vi "Improved find target.vi"(9 "robot location":dbl[](array[numeric]), 10 "Dispaly map":u16[][](array[ring])) -> (2 "target location":dbl[](array[numeric]))   [LabVIEW 2015]
panel:
  out "points":dbl
  out "Highest priority locations":i32[][](array[numeric])
  out "distances":dbl[](array[numeric])
  out "Priority map":dbl[][](array[numeric])
  out "x":dbl
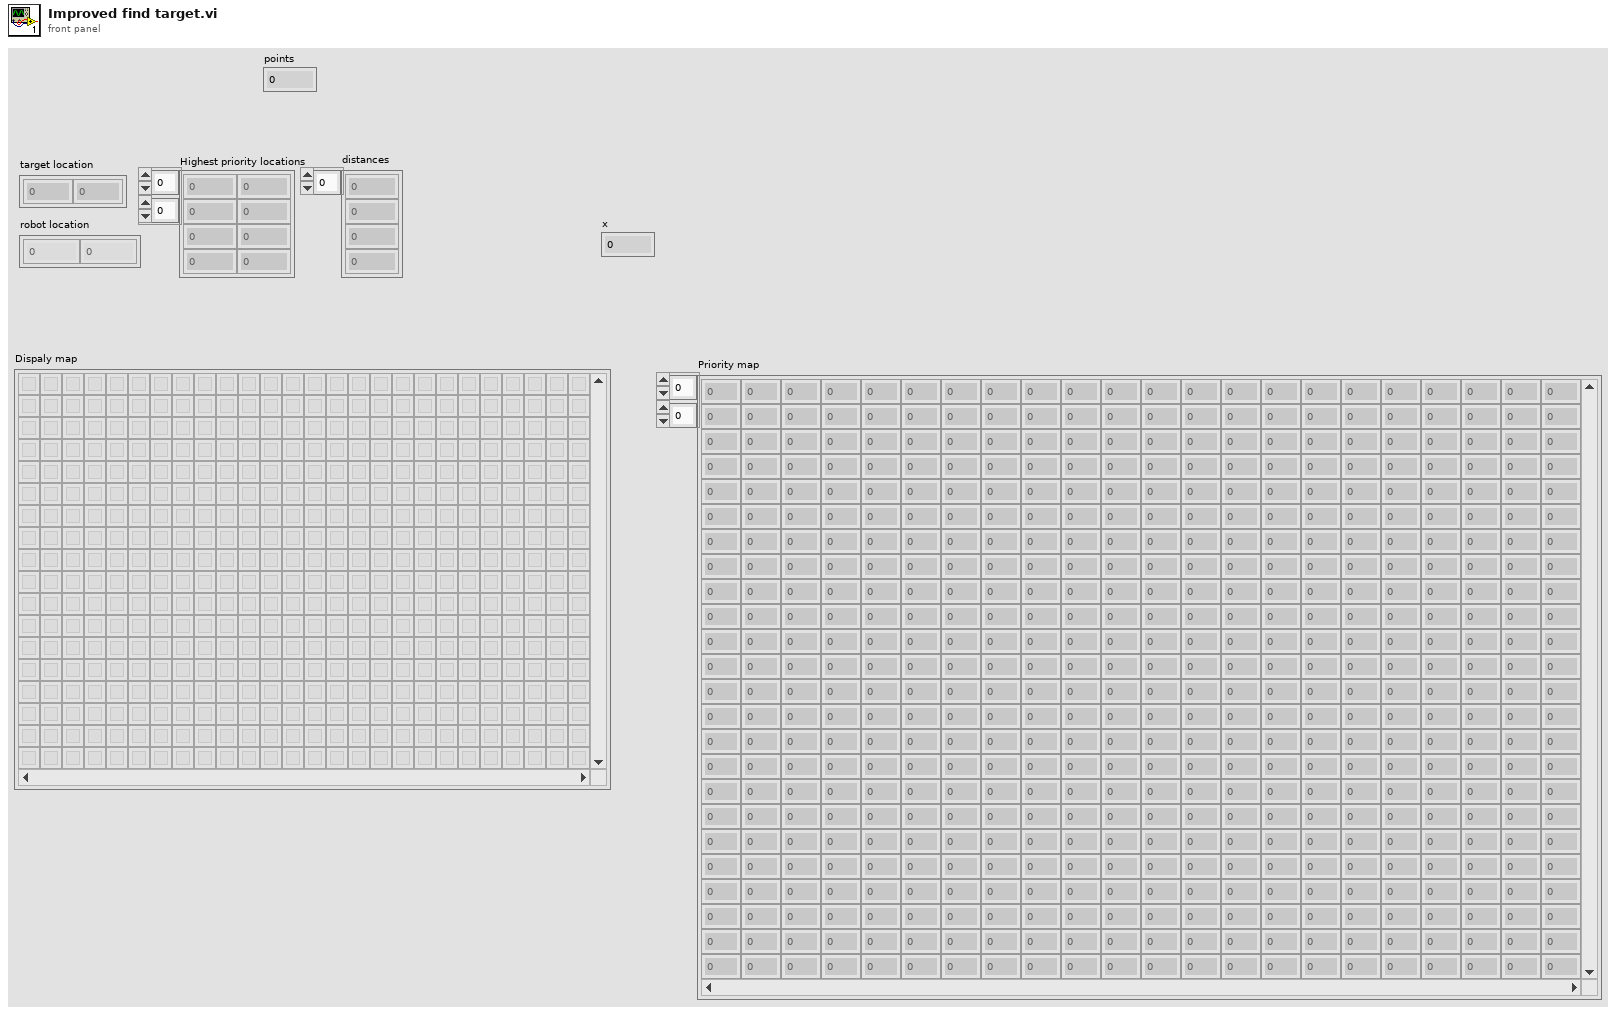
[diagram p1: front panel]
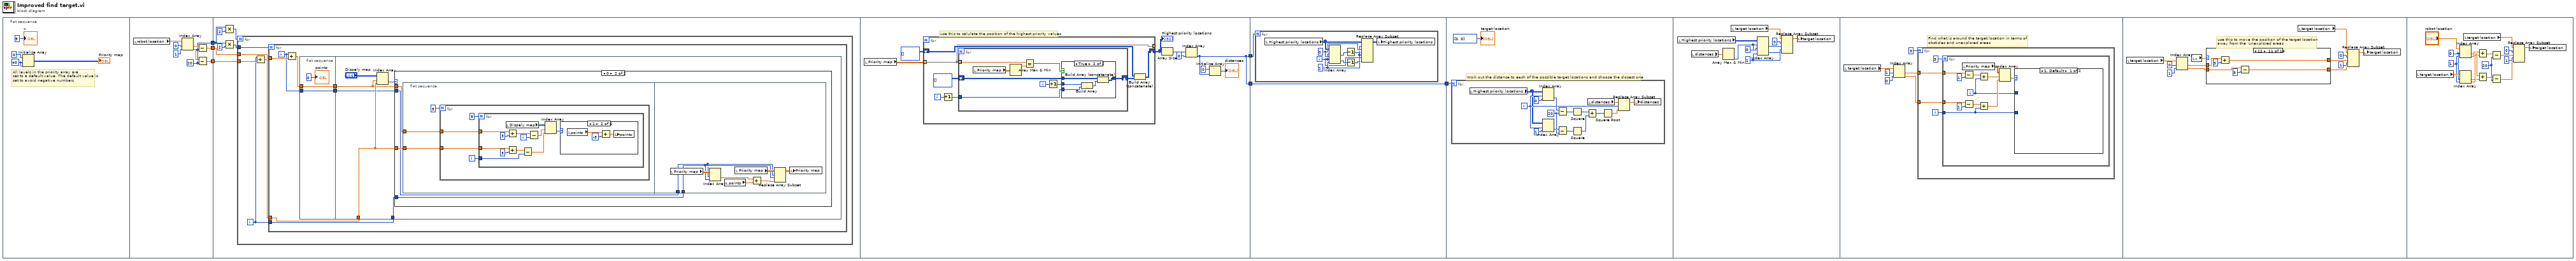
[diagram p0: block diagram]
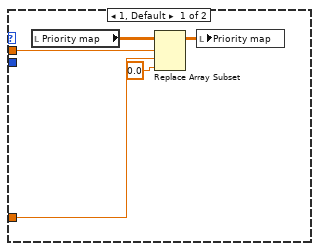
[diagram p2: hidden frame]
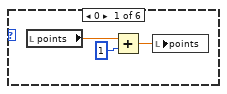
[diagram p3: hidden frame]
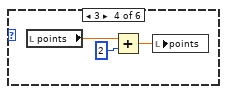
[diagram p5: hidden frame]
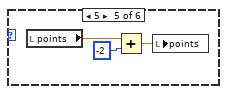
[diagram p6: hidden frame]
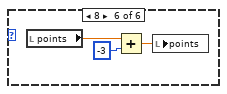
[diagram p7: hidden frame]
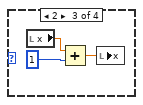
[diagram p12: hidden frame]
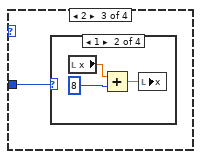
[diagram p14: hidden frame]
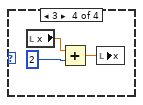
[diagram p17: hidden frame]
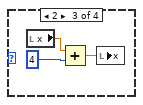
[diagram p20: hidden frame]
diagram:
  n1 = flat-sequence {
    tunnel: [w15] -> w3
    tunnel: [w14] -> w2
    tunnel: [w11] -> w1
    tunnel: w3 -> [w25]
    tunnel: w2 -> [w24]
    tunnel: w1 -> [w19]
    tunnel: [w98] -> w6
    tunnel: [w98] -> w5
    tunnel: w6 -> [w129]
    tunnel: [w129] -> w4
    tunnel: w5 -> [w128]
    tunnel: w4 -> [w139]
    frame #0 {
      w7 = 40
      # "All levels in the priority array are \nset to a default value. The default value is \nset to avoid negative numbers"
      n2 = Initialize Array(0, w7, w7) -> (→"Priority map":i32[][])
      "x" <- 5
    }
    frame #1 {
      w11 = 20
      n3 = local read "robot location"() -> (w16:dbl[])
      n4 = Index Array(array=w16, index #1=0, index #2=1) -> (element #1=w12:dbl, element #2=w13:dbl)
      n5 = Subtract(x=w12, y=w11) -> (x-y=w15:dbl)
      n6 = Subtract(x=w13, y=w11) -> (x-y=w14:dbl)
    }
    frame #2 {
      n7 = Multiply(x=w19, y=2) -> (x*y=w23:i32)
      n8 = Multiply(x=w19, y=2) -> (x*y=w21:i32)
      n9 = for {
        N: w23 -> [_]
        tunnel: w21 -> [w30]
        tunnel: w24 -> [w29]
        tunnel: w25 -> [w27]
        i -> [w26]
        n10 = Add(x=w26, y=w29) -> (x+y=w28:dbl)
        n11 = for {
          N: w30 -> [_]
          tunnel: w28 -> [w37]
          tunnel: w27 -> [w35]
          tunnel: w26 -> [w33]
          i -> [w31]
          n12 = Add(x=w31, y=w35) -> (x+y=w34:dbl)
          n13 = flat-sequence {
            tunnel: w34 -> [w40]
            tunnel: [w40] -> w36
            tunnel: [w38] -> w32
            tunnel: w31 -> [w38]
            tunnel: w37 -> [w46]
            tunnel: w36 -> [w45]
            tunnel: w33 -> [w42]
            tunnel: w32 -> [w41]
            frame #0 {
              "points" <- 0
            }
            frame #1 {
              n14 = Index Array(array="Dispaly map", index (row)=w45, index (col)=w46) -> (element=w43:u16)
              n15 = case shown="0" w43 {
                tunnel: w46 -> [w48 w55]
                tunnel: w45 -> [w47 w54]
                tunnel: w42 -> [_ w53]
                tunnel: w41 -> [_ w52]
                frame 1, Default {
                  n16 = local read "Priority map"() -> (w51:dbl[][])
                  n17 = Replace Array Subset(array=w51, new element=0.0, index (row)=w47, index (col)=w48) -> (w50:dbl[][])
                  n18 = local write "Priority map"(w50) -> ()
                }
                frame 0 {
                  n19 = flat-sequence {
                    tunnel: w55 -> [w58]
                    tunnel: w54 -> [w57]
                    tunnel: w53 -> [w92]
                    tunnel: w52 -> [w91]
                    frame #0 {
                      n20 = for {
                        N: 5 -> [_]
                        tunnel: w58 -> [w62]
                        tunnel: w57 -> [w61]
                        i -> [w59]
                        n21 = for {
                          N: 5 -> [_]
                          tunnel: w62 -> [w71]
                          tunnel: w61 -> [w64]
                          tunnel: w59 -> [w67]
                          i -> [w69]
                          n22 = local read "Dispaly map"() -> (w74:u16[][])
                          n23 = Add(x=w64, y=3) -> (x+y=w70:dbl)
                          n24 = Add(x=w71, y=3) -> (x+y=w68:dbl)
                          n25 = Subtract(x=w68, y=w67) -> (x-y=w66:dbl)
                          n26 = Subtract(x=w70, y=w69) -> (x-y=w65:dbl)
                          n27 = Index Array(array=w74, index (row)=w65, index (col)=w66) -> (element=w63:u16)
                          n28 = case shown="1" w63 {
                            frame 0 {
                              n29 = local read "points"() -> (w75:dbl)
                              n30 = Add(x=w75, y=1) -> (x+y=w76:dbl)
                              n31 = local write "points"(w76) -> ()
                            }
                            frame 1 {
                              n32 = local read "points"() -> (w79:dbl)
                              n33 = Add(x=w79, y=-3) -> (x+y=w78:dbl)
                              n34 = local write "points"(w78) -> ()
                            }
                            frame 2, Default {
                            }
                            frame 3 {
                              n35 = local read "points"() -> (w81:dbl)
                              n36 = Add(x=w81, y=2) -> (x+y=w82:dbl)
                              n37 = local write "points"(w82) -> ()
                            }
                            frame 5 {
                              n38 = local read "points"() -> (w84:dbl)
                              n39 = Add(x=w84, y=-2) -> (x+y=w85:dbl)
                              n40 = local write "points"(w85) -> ()
                            }
                            frame 8 {
                              n41 = local read "points"() -> (w87:dbl)
                              n42 = Add(x=w87, y=-3) -> (x+y=w88:dbl)
                              n43 = local write "points"(w88) -> ()
                            }
                          }
                        }
                      }
                    }
                    frame #1 {
                      n44 = local read "Priority map"() -> (w93:dbl[][])
                      n45 = Index Array(array=w93, index (row)=w91, index (col)=w92) -> (element=w96:dbl)
                      n46 = local read "points"() -> (w90:dbl)
                      n47 = local read "Priority map"() -> (w94:dbl[][])
                      n48 = Add(x=w96, y=w90) -> (x+y=w97:dbl)
                      n49 = Replace Array Subset(array=w94, new element=w97, index (row)=w91, index (col)=w92) -> (w95:dbl[][])
                      n50 = local write "Priority map"(w95) -> ()
                    }
                  }
                }
              }
            }
          }
        }
      }
    }
    frame #3 {
      # "use this to calulate the position of the highest priority values"
      n51 = local read "Priority map"() -> (w104:dbl[][])
      n52 = for {
        tunnel: w104 -> [w107] mode=indexing
        shift-right: [w110] -> w101
        shift-left: i32[][] [] -> [w108]
        tunnel: [w107] -> _ mode=indexing
        i -> [w112]
        n53 = Increment(x=w112) -> (x+1=w111:i32)
        n54 = for {
          tunnel: w107 -> [w121] mode=indexing
          tunnel: w111 -> [w117]
          shift-right: [w116] -> w109
          shift-left: i32[][] [] -> [w115]
          i -> [w119]
          n55 = local read "Priority map"() -> (w113:dbl[][])
          n56 = Array Max & Min(array=w113) -> (max value=w114:dbl)  [unwired: 3 out]
          n57 = Equal?(x=w121, y=w114) -> (x = y?=w120:bool)
          n58 = Increment(x=w119) -> (x+1=w118:i32)
          n59 = case shown="True" w120 {
            tunnel: w118 -> [_ w127]
            tunnel: w117 -> [_ w126]
            tunnel: [w122 w124] -> w116
            tunnel: w115 -> [w122 w123]
            frame False {
            }
            frame True {
              n60 = Build Array(w127, w126) -> (w125:i32[])
              n61 = Build Array (concatenate)(w123, w125) -> (w124:i32[][])
            }
          }
        }
        n62 = Build Array (concatenate)(w108, w109) -> (w110:i32[][])
      }
      "Highest priority locations" <- w101
      n63 = Array Size(array=w101) -> (size(s)=w100:i32[])
      n64 = Index Array(array=w100, index=0) -> (element=w98:i32)
      n65 = Initialize Array(0, w98) -> (→"distances":i32[])
    }
    frame #4 {
      n66 = for {
        N: w128 -> [_]
        i -> [w132]
        w134 = 1
        w133 = 0
        n67 = local read "Highest priority locations"() -> (w136:i32[][])
        n68 = Index Array(array=w136, index (row) #1=w132, index (col) #1=w133, index (row) #2=w132, index (col) #2=w134) -> (element #1=w138:i32, element #2=w137:i32)
        n69 = Decrement(x=w138) -> (x-1=w131:i32)
        n70 = Decrement(x=w137) -> (x-1=w130:i32)
        n71 = Replace Array Subset(array=w136, new element #1=w131, index (row) #1=w132, index (col) #1=w133, new element #2=w130, index (row) #2=w132, index (col) #2=w134) -> (w135:i32[][])
        n72 = local write "Highest priority locations"(w135) -> ()
      }
    }
    frame #5 {
      # "Work out the distance to each of the possible target locations and choose the closest one"
      n73 = for {
        N: w139 -> [_]
        i -> [w145]
        w141 = 20
        n74 = local read "Highest priority locations"() -> (w144:i32[][])
        n75 = Index Array(array=w144, index (row)=w145, index (col)=0) -> (element=w155:i32)
        n76 = Index Array(array=w144, index (row)=w145, index (col)=1) -> (element=w154:i32)
        n77 = Subtract(x=w155, y=w141) -> (x-y=w153:i32)
        n78 = Subtract(x=w154, y=w141) -> (x-y=w148:i32)
        n79 = Square(x=w153) -> (x^2=w151:i32)
        n80 = Square(x=w148) -> (x^2=w152:i32)
        n81 = Add(x=w151, y=w152) -> (x+y=w150:i32)
        n82 = local read "distances"() -> (w142:dbl[])
        n83 = Square Root(x=w150) -> (sqrt(x)=w149:dbl)
        n84 = Replace Array Subset(array=w142, new element=w149, index=w145) -> (w143:dbl[])
        n85 = local write "distances"(w143) -> ()
      }
      "target location" <- i32[] [0, 0]
    }
    frame #6 {
      w158 = 1
      n86 = local read "Highest priority locations"() -> (w160:i32[][])
      n87 = local read "distances"() -> (w165:dbl[])
      n88 = Array Max & Min(array=w165) -> (min index (indices)=w159:i32)  [unwired: 3 out]
      n89 = local read "target location"() -> (w163:dbl[])
      n90 = Index Array(array=w160, index (row) #1=w159, index (col) #1=0, index (row) #2=w159, index (col) #2=w158) -> (element #1=w157:i32, element #2=w156:i32)
      n91 = Replace Array Subset(array=w163, new element #1=w157, index #1=0, new element #2=w156, index #2=w158) -> (w164:dbl[])
      n92 = local write "target location"(w164) -> ()
    }
    frame #7 {
      # "Find what is around the target location in terms of \nobsticles and unexplored areas"
      n93 = local read "target location"() -> (w171:dbl[])
      n94 = Index Array(array=w171, index #1=1, index #2=0) -> (element #1=w167:dbl, element #2=w166:dbl)
      n95 = for {
        N: 3 -> [_]
        tunnel: w167 -> [w174]
        tunnel: w166 -> [w173]
        i -> [w172]
        n96 = for {
          N: 3 -> [_]
          tunnel: w174 -> [w184]
          tunnel: w173 -> [w183]
          tunnel: w172 -> [w177]
          i -> [w178]
          n97 = local read "Priority map"() -> (w187:dbl[][])
          n98 = Subtract(x=w184, y=1) -> (x-y=w182:dbl)
          n99 = Subtract(x=w183, y=1) -> (x-y=w181:dbl)
          n100 = Add(x=w182, y=w178) -> (x+y=w180:dbl)
          n101 = Add(x=w181, y=w177) -> (x+y=w179:dbl)
          n102 = Index Array(array=w187, index (row)=w180, index (col)=w179) -> (element=w176:dbl)
          n103 = case shown="1, Default" w176 {
            tunnel: w178 -> [_ w189]
            tunnel: w177 -> [_ w188]
            frame 1, Default {
            }
            frame 0 {
              n104 = case shown="1" w189 {
                tunnel: w188 -> [_ w190 w194 w201]
                frame 0, Default {
                }
                frame 1 {
                  n105 = case shown="1" w190 {
                    frame 0, Default {
                    }
                    frame 1 {
                    }
                    frame 2 {
                      n106 = local read "x"() -> (w193:dbl)
                      n107 = Add(x=w193, y=1) -> (x+y=w192:dbl)
                      n108 = local write "x"(w192) -> ()
                    }
                    frame 3 {
                    }
                  }
                }
                frame 2 {
                  n109 = case shown="1" w194 {
                    frame 0, Default {
                    }
                    frame 1 {
                      n110 = local read "x"() -> (w197:dbl)
                      n111 = Add(x=w197, y=8) -> (x+y=w196:dbl)
                      n112 = local write "x"(w196) -> ()
                    }
                    frame 2 {
                    }
                    frame 3 {
                      n113 = local read "x"() -> (w200:dbl)
                      n114 = Add(x=w200, y=2) -> (x+y=w199:dbl)
                      n115 = local write "x"(w199) -> ()
                    }
                  }
                }
                frame 3 {
                  n116 = case shown="1" w201 {
                    frame 0, Default {
                    }
                    frame 1 {
                    }
                    frame 2 {
                      n117 = local read "x"() -> (w204:dbl)
                      n118 = Add(x=w204, y=4) -> (x+y=w203:dbl)
                      n119 = local write "x"(w203) -> ()
                    }
                    frame 3 {
                    }
                  }
                }
              }
            }
          }
        }
      }
    }
    frame #8 {
      # "use this to move the position of the target location\naway from the  unexplored areas"
      n120 = local read "target location"() -> (w213:dbl[])
      n121 = Index Array(array=w213, index #1=0, index #2=1) -> (element #1=w206:dbl, element #2=w205:dbl)
      n122 = local read "x"() -> (w216:dbl)
      n123 = case shown="12" w216 {
        tunnel: [w217 w221 w225 w230 w236 w241 w244 w249 w252 w258 w264 w270 w271 w277 w285 w290] -> w208
        tunnel: [w218 w220 w226 w231 w237 w242 w243 w250 w253 w257 w265 w269 w272 w279 w286 w291] -> w207
        tunnel: w206 -> [w218 w219 w227 w232 w238 w242 w246 w250 w254 w260 w266 w269 w276 w280 w287 w292]
        tunnel: w205 -> [w217 w222 w225 w229 w235 w241 w245 w249 w251 w259 w263 w270 w275 w278 w284 w289]
        frame 0, Default {
        }
        frame 1 {
          n124 = Add(x=w219, y=0) -> (x+y=w220:dbl)
          n125 = Add(x=w222, y=3) -> (x+y=w221:dbl)
        }
        frame 2 {
          n126 = Subtract(x=w227, y=3) -> (x-y=w226:dbl)
        }
        frame 3 {
          n127 = Subtract(x=w232, y=3) -> (x-y=w231:dbl)
          n128 = Add(x=w229, y=3) -> (x+y=w230:dbl)
        }
        frame 4 {
          n129 = Add(x=w238, y=0) -> (x+y=w237:dbl)
          n130 = Subtract(x=w235, y=3) -> (x-y=w236:dbl)
        }
        frame 5 {
        }
        frame 6 {
          n131 = Subtract(x=w246, y=3) -> (x-y=w243:dbl)
          n132 = Subtract(x=w245, y=3) -> (x-y=w244:dbl)
        }
        frame 7 {
        }
        frame 8 {
          n133 = Add(x=w254, y=3) -> (x+y=w253:dbl)
          n134 = Add(x=w251, y=0) -> (x+y=w252:dbl)
        }
        frame 9 {
          n135 = Add(x=w260, y=3) -> (x+y=w257:dbl)
          n136 = Add(x=w259, y=3) -> (x+y=w258:dbl)
        }
        frame 12 {
          n137 = Add(x=w266, y=3) -> (x+y=w265:dbl)
          n138 = Subtract(x=w263, y=3) -> (x-y=w264:dbl)
        }
        frame 14 {
        }
        frame 20 {
          n139 = Add(x=w276, y=3) -> (x+y=w272:dbl)
          n140 = Add(x=w275, y=3) -> (x+y=w271:dbl)
        }
        frame 30 {
          n141 = Subtract(x=w280, y=3) -> (x-y=w279:dbl)
          n142 = Add(x=w278, y=3) -> (x+y=w277:dbl)
        }
        frame 40 {
          n143 = Add(x=w287, y=3) -> (x+y=w286:dbl)
          n144 = Subtract(x=w284, y=3) -> (x-y=w285:dbl)
        }
        frame 50 {
          n145 = Subtract(x=w292, y=3) -> (x-y=w291:dbl)
          n146 = Subtract(x=w289, y=3) -> (x-y=w290:dbl)
        }
      }
      n147 = local read "target location"() -> (w215:dbl[])
      n148 = Replace Array Subset(array=w215, new element #1=w207, index #1=0, new element #2=w208, index #2=1) -> (w214:dbl[])
      n149 = local write "target location"(w214) -> ()
    }
    frame #9 {
      w301 = 20
      w308 = 1
      w309 = 0
      n150 = local read "target location"() -> (w310:dbl[])
      n151 = Index Array(array="robot location", index #1=w309, index #2=w308) -> (element #1=w306:dbl, element #2=w307:dbl)
      n152 = Index Array(array=w310, index #1=w309, index #2=w308) -> (element #1=w304:dbl, element #2=w305:dbl)
      n153 = local read "target location"() -> (w298:dbl[])
      n154 = Add(x=w307, y=w305) -> (x+y=w303:dbl)
      n155 = Add(x=w306, y=w304) -> (x+y=w302:dbl)
      n156 = Subtract(x=w303, y=w301) -> (x-y=w300:dbl)
      n157 = Subtract(x=w302, y=w301) -> (x-y=w295:dbl)
      n158 = Replace Array Subset(array=w298, new element #1=w300, index #1=0, new element #2=w295, index #2=1) -> (w299:dbl[])
      n159 = local write "target location"(w299) -> ()
    }
  }
